vi "Autonomous Independent.vi"   [LabVIEW 2013]
doc: "This VI is called when autonomous begins, and will automatically be terminated when autonomous ends. You can carry out timed or sensor driven robot movement independently without needing to return to the caller."
uses:
  <vilib>/Rock Robotics/WPI/Solenoid/WPI_SolenoidValue.ctl
  Robot Global Data.vi
  <vilib>/Rock Robotics/WPI/Solenoid/Deprecated/WPI_SolenoidGetBool.vi
  <vilib>/Rock Robotics/WPI/Solenoid/WPI_SolenoidSetEnum.vi
  <vilib>/Rock Robotics/WPI/RobotDrive/WPI_RobotDriveGetSetRefNum.vi
  <vilib>/Rock Robotics/WPI/RobotDrive/WPI_RobotDriveArcadeDrive_Standard(NoSaturation).vi
  <vilib>/Rock Robotics/WPI/Joystick/WPI_JoystickGetSetRefNum.vi
panel:
  # "Be sure to right-click and choose Data Operations>>Make Current Value default if you want to save the array values with the VI"
types:
  T1 = typedef "WPI_JoystickDevRef.ctl" = cluster{"Device":T2}
  T2 = typedef "WPI_JoystickDeviceEnum.ctl" = enum16{"USB 1", "USB 2", "USB 3", "USB 4", "Kinect 1", "Kinect 2"}
  T3 = typedef "WPI_SolenoidDevRef.ctl" = cluster{"DevStatus":errorcluster, "Solenoid Module":T4, "Forward Solenoid Channel":T5, "Reverse Solenoid Channel":T5}
  T4 = typedef "FPGA_TypedefSolenoidModule.ctl" = enum16{"Solenoid Module 1", "Solenoid Module 2"}
  T5 = typedef "WPI_SolenoidChannel.ctl" = enum8{"Solenoid 1", "Solenoid 2", "Solenoid 3", "Solenoid 4", "Solenoid 5", "Solenoid 6", "Solenoid 7", "Solenoid 8", "Invalid"}
  T6 = typedef "WPI_SolenoidValue.ctl" = enum16{"Off", "On", "Forward", "Reverse"}
  T7 = typedef "WPI_RobotDriveDevRef.ctl" = cluster{"DevStatus":errorcluster, "Motors[]":T8[], "Square Inputs":bool, "Max Output":dbl, "Isochronous":bool}
  T8 = typedef "WPI_MotorControlDeviceRef.ctl" = cluster{"DeviceStatus":errorcluster, "Type":enum16{"PWM", "CAN"}, "PWM":cluster{"Digital Module":T9, "PWM Channel":T10, "DeadBand":T11}, "CAN":cluster{"Device Number":u8, "Control Mode":T12, "Semaphore":T13, "Max Vout":dbl}, "Invert":bool, "TransformRef":T14, "InvTransformRef":T14}
  T9 = typedef "FPGA_TypedefDigitalModule.ctl" = enum16{"Digital Module 1", "Digital Module 2"}
  T10 = typedef "FPGA_DIOPWMChannel.ctl" = enum8{"PWM 1", "PWM 2", "PWM 3", "PWM 4", "PWM 5", "PWM 6", "PWM 7", "PWM 8", "PWM 9", "PWM 10", "Invalid"}
  T11 = typedef "WPI_PWMDeadband.ctl" = cluster{"Name":string, "maxPositivePwm":i32, "minPositivePwm":i32, "centerPwm":i32, "maxNegativePwm":i32, "minNegativePwm":i32, "angularRange":u16}
  T12 = typedef "WPI_CANJaguar_ControlMode.ctl" = enum8{"Percent VBus", "Current", "Speed", "Position", "Voltage"}
  T13 = typedef "Semaphore RefNum" = refnum<k1>
  T14 = typedef "WPI_PWMTransform_ConPane.ctl" = refnum<vi>
  T15 = cluster{"axis 1 (x)":dbl, "axis 2 (y)":dbl, "axis 3 (throttle)":dbl, "axis 4":dbl, "axis 5":dbl, "axis 6":dbl}
  T16 = typedef "WPI_DigitalInputDevRef.ctl" = cluster{"DevStatus":errorcluster, "DIO Channel":T17, "Digital Module":T9}
  T17 = typedef "FPGA_DIOChannel.ctl" = enum8{"DIO 1", "DIO 2", "DIO 3", "DIO 4", "DIO 5", "DIO 6", "DIO 7", "DIO 8", "DIO 9", "DIO 10", "DIO 11", "DIO 12", "DIO 13", "DIO 14", "Invalid"}
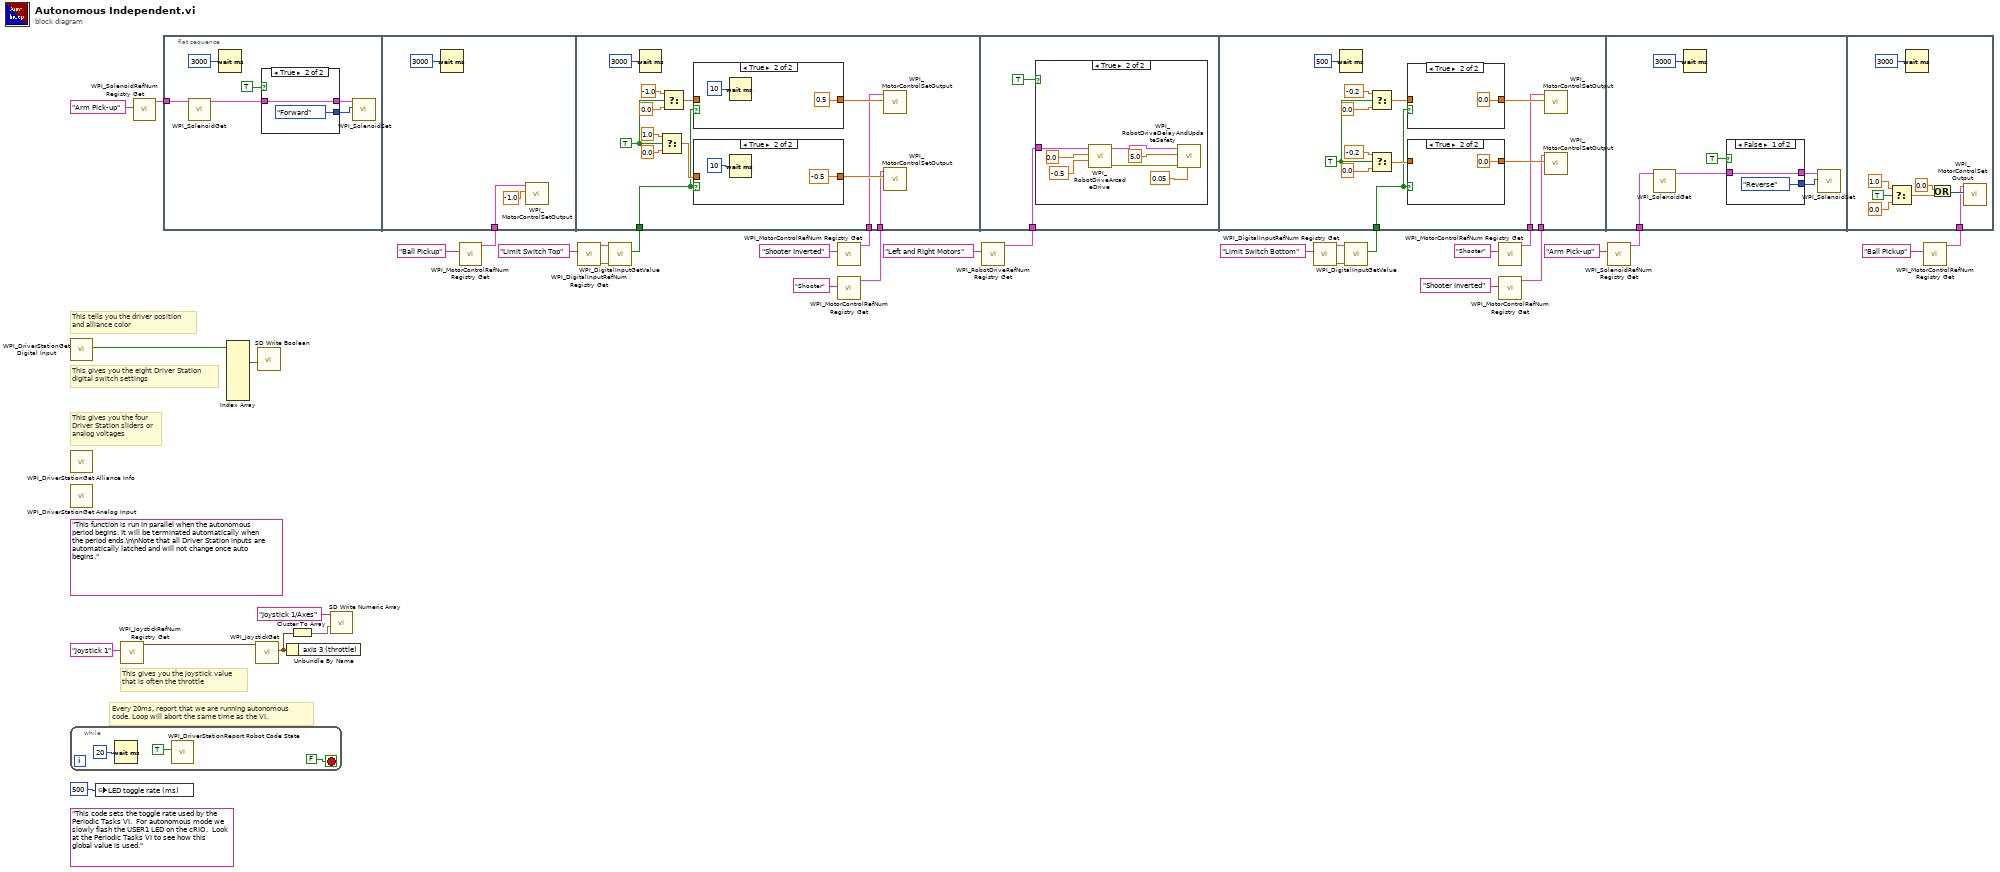
[diagram p0: block diagram]
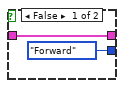
[diagram p2: hidden frame]
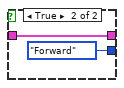
[diagram p8: hidden frame]
diagram:
  (unwired) "This code sets the toggle rate used by the Periodic Tasks VI.  For autonomous mode we slowly flash the USER1 LED on the cRIO.  Look at the Periodic Tasks VI to see how this global value is used."
  (unwired) "This function is run in parallel when the autonomous period begins. It will be terminated automatically when the period ends.\n\nNote that all Driver Station inputs are automatically latched and will not change once auto begins."
  # "Every 20ms, report that we are running autonomous\ncode. Loop will abort the same time as the VI."
  # "This gives you the joystick value\nthat is often the throttle"
  # "This tells you the driver position\nand alliance color"
  # "This gives you the eight Driver Station\ndigital switch settings"
  # "This gives you the four\nDriver Station sliders or\nanalog voltages"
  n1 = call <vilib>:"WPI_DriverStationGet Digital Input.vi"() -> ("Driver Station Digital Input (1-8)"=w34:bool[])  [unwired: 11 out]
  n2 = call <vilib>:"WPI_DriverStationGet Alliance Info.vi"() -> ()  [unwired: 12 out]
  n3 = call <vilib>:"WPI_DriverStationGet Analog Input.vi"() -> ()  [unwired: 12 out]
  n4 = while {
    stop <- FALSE stop-if-true
    n5 = Wait (ms)(milliseconds to wait=u32 20) -> ()  [unwired: 1 out]
    n6 = call <vilib>:"WPI_DriverStationReport Robot Code State.vi"("Autonomous"=TRUE) -> ()  [unwired: 10 in, 1 out]
  }
  n7 = global write "Robot Global Data.vi" "LED toggle rate (ms)"(u32 500 ("LED ms toggle rate")) -> ()
  n8 = call <vilib>:"WPI_JoystickRefNum Registry Get.vi"("refnum name"="Joystick 1") -> ("JoystickDevRef"=w32:T1)  [unwired: 1 in, 9 out]
  n9 = call <vilib>:"WPI_SolenoidRefNum Registry Get.vi"("refnum name"="Arm Pick-up") -> ("SolenoidDevRef"=w9:T3)  [unwired: 9 in, 1 out]
  n10 = flat-sequence {
    tunnel: w9 -> [w38]
    tunnel: w15 -> [w49]
    tunnel: w18 -> [w53]
    tunnel: w13 -> [w52]
    tunnel: w11 -> [w51]
    tunnel: w17 -> [w70]
    tunnel: w22 -> [w81]
    tunnel: w7 -> [w80]
    tunnel: w5 -> [w79]
    tunnel: w3 -> [w96]
    tunnel: w1 -> [w106]
    frame #0 {
      n11 = call-poly <vilib>:"WPI_SolenoidGet.vi"("SolenoidDevRef"=w38) -> ("SolenoidDevRef"=w43:T3)  [unwired: 8 in, 2 out]
      n12 = Wait (ms)(milliseconds to wait=u32 3000) -> ()  [unwired: 1 out]
      n13 = case shown="True" TRUE {
        tunnel: w43 -> [w44 w47]
        tunnel: [w44 w47] -> w42
        tunnel: [WPI_SolenoidValue."Forward" ("Value") WPI_SolenoidValue."Forward" ("Value")] -> w41
        frame False {
        }
        frame True {
        }
      }
      n14 = call-poly <vilib>:"WPI_SolenoidSet.vi"("Value"=w41, "SolenoidDevRef"=w42) -> ()  [unwired: 8 in, 2 out]
    }
    frame #1 {
      n15 = Wait (ms)(milliseconds to wait=u32 3000) -> ()  [unwired: 1 out]
      n16 = call <vilib>:"WPI_MotorControlSetOutput.vi"("Output"=-1.0, "MotorControlDevRef"=w49) -> ()  [unwired: 7 in, 3 out]
    }
    frame #2 {
      w57 = TRUE
      n17 = Wait (ms)(milliseconds to wait=u32 3000) -> ()  [unwired: 1 out]
      n18 = Select(t=1.0, s=w57, f=0.0) -> (s? t:f=w63:dbl)
      n19 = Select(t=-1.0, s=w57, f=0.0) -> (s? t:f=w60:dbl)
      n20 = case shown="True" w53 {
        tunnel: [w64 0.5 ("f")] -> w58
        tunnel: w60 -> [w64 _]
        frame False {
        }
        frame True {
          n21 = Wait (ms)(milliseconds to wait=u32 10) -> ()  [unwired: 1 out]
        }
      }
      n22 = case shown="True" w53 {
        tunnel: [w67 -0.5 ("f")] -> w61
        tunnel: w63 -> [w67 _]
        frame False {
        }
        frame True {
          n23 = Wait (ms)(milliseconds to wait=u32 10) -> ()  [unwired: 1 out]
        }
      }
      n24 = call <vilib>:"WPI_MotorControlSetOutput.vi"("Output"=w58, "MotorControlDevRef"=w52) -> ()  [unwired: 7 in, 3 out]
      n25 = call <vilib>:"WPI_MotorControlSetOutput.vi"("Output"=w61, "MotorControlDevRef"=w51) -> ()  [unwired: 7 in, 3 out]
    }
    frame #3 {
      n26 = case shown="True" TRUE {
        tunnel: w70 -> [_ w78]
        frame False {
        }
        frame True {
          n27 = call-poly <vilib>:"WPI_RobotDriveArcadeDrive.vi"("Y axis value"=-0.5, "X axis value"=0.0, "RobotDriveDevRef"=w78) -> ("error out"=w75:errorcluster, "RobotDriveDevRef"=w74:T7)  [unwired: 6 in, 1 out]
          n28 = call <vilib>:"WPI_RobotDriveDelayAndUpdateSafety.vi"("Feed time (s)"=0.05, "error in (no error)"=w75, "Delay (s)"=5.0, "RobotDriveDevRef"=w74) -> ()  [unwired: 6 in, 2 out]
        }
      }
    }
    frame #4 {
      w82 = TRUE
      n29 = Wait (ms)(milliseconds to wait=u32 500) -> ()  [unwired: 1 out]
      n30 = Select(t=-0.2, s=w82, f=0.0) -> (s? t:f=w84:dbl)
      n31 = Select(t=-0.2, s=w82, f=0.0) -> (s? t:f=w83:dbl)
      n32 = case shown="True" w81 {
        tunnel: [w94 0.0 ("f")] -> w89
        tunnel: w84 -> [w94 _]
        frame False {
        }
        frame True {
        }
      }
      n33 = case shown="True" w81 {
        tunnel: [w92 0.0 ("f")] -> w86
        tunnel: w83 -> [w92 _]
        frame False {
        }
        frame True {
        }
      }
      n34 = call <vilib>:"WPI_MotorControlSetOutput.vi"("Output"=w89, "MotorControlDevRef"=w79) -> ()  [unwired: 7 in, 3 out]
      n35 = call <vilib>:"WPI_MotorControlSetOutput.vi"("Output"=w86, "MotorControlDevRef"=w80) -> ()  [unwired: 7 in, 3 out]
    }
    frame #5 {
      n36 = call-poly <vilib>:"WPI_SolenoidGet.vi"("SolenoidDevRef"=w96) -> ("SolenoidDevRef"=w101:T3)  [unwired: 8 in, 2 out]
      n37 = Wait (ms)(milliseconds to wait=u32 3000) -> ()  [unwired: 1 out]
      n38 = case shown="False" TRUE {
        tunnel: w101 -> [w102 w105]
        tunnel: [w102 w105] -> w100
        tunnel: [WPI_SolenoidValue."Reverse" ("Value") WPI_SolenoidValue."Forward" ("Value")] -> w99
        frame False {
        }
        frame True {
        }
      }
      n39 = call-poly <vilib>:"WPI_SolenoidSet.vi"("Value"=w99, "SolenoidDevRef"=w100) -> ()  [unwired: 8 in, 2 out]
    }
    frame #6 {
      n40 = Select(t=1.0, s=TRUE, f=0.0) -> (s? t:f=w110:dbl)
      n41 = Wait (ms)(milliseconds to wait=u32 3000) -> ()  [unwired: 1 out]
      n42 = Or(x=0.0, y=w110) -> (x .or. y?=w109:i32)
      n43 = call <vilib>:"WPI_MotorControlSetOutput.vi"("Output"=w109, "MotorControlDevRef"=w106) -> ()  [unwired: 7 in, 3 out]
    }
  }
  n44 = Index Array(array=w34) -> (element #2=w27:bool)  [unwired: 8 in, 7 out]
  n45 = call <vilib>:"WPI_JoystickGet.vi"("JoystickDevRef"=w32) -> ("Axes"=w29:T15)  [unwired: 1 in, 5 out]
  n46 = call <vilib>:"SD Write Boolean.vi"("Boolean"=w27) -> ()  [unwired: 9 in, 2 out]
  n47 = Unbundle By Name(w29) -> ()  [unwired: 1 out]
  n48 = Cluster To Array(cluster=w29) -> (array=w30:dbl[])
  n49 = call <vilib>:"SD Write Numeric Array.vi"("Numeric Array"=w30, "Name"="Joystick 1/Axes") -> ()  [unwired: 8 in, 2 out]
  n50 = call <vilib>:"WPI_MotorControlRefNum Registry Get.vi"("refnum name"="Ball Pickup") -> ("MotorControlDevRef"=w15:T8)  [unwired: 9 in, 1 out]
  n51 = call <vilib>:"WPI_DigitalInputRefNum Registry Get.vi"("refnum name"="Limit Switch Top") -> ("error out"=w20:errorcluster, "DigitalInputDevRef"=w21:T16)  [unwired: 9 in]
  n52 = call <vilib>:"WPI_DigitalInputGetValue.vi"("error in (no error)"=w20, "DigitalInputDevRef"=w21) -> ("Value"=w18:bool)  [unwired: 7 in, 2 out]
  n53 = call <vilib>:"WPI_MotorControlRefNum Registry Get.vi"("refnum name"="Shooter Inverted") -> ("MotorControlDevRef"=w13:T8)  [unwired: 9 in, 1 out]
  n54 = call <vilib>:"WPI_MotorControlRefNum Registry Get.vi"("refnum name"="Shooter") -> ("MotorControlDevRef"=w11:T8)  [unwired: 9 in, 1 out]
  n55 = call <vilib>:"WPI_RobotDriveRefNum Registry Get.vi"("refnum name"="Left and Right Motors") -> ("RobotDriveDevRef"=w17:T7)  [unwired: 9 in, 1 out]
  n56 = call <vilib>:"WPI_DigitalInputRefNum Registry Get.vi"("refnum name"="Limit Switch Bottom") -> ("error out"=w24:errorcluster, "DigitalInputDevRef"=w25:T16)  [unwired: 9 in]
  n57 = call <vilib>:"WPI_DigitalInputGetValue.vi"("error in (no error)"=w24, "DigitalInputDevRef"=w25) -> ("Value"=w22:bool)  [unwired: 7 in, 2 out]
  n58 = call <vilib>:"WPI_MotorControlRefNum Registry Get.vi"("refnum name"="Shooter") -> ("MotorControlDevRef"=w5:T8)  [unwired: 9 in, 1 out]
  n59 = call <vilib>:"WPI_MotorControlRefNum Registry Get.vi"("refnum name"="Shooter Inverted") -> ("MotorControlDevRef"=w7:T8)  [unwired: 9 in, 1 out]
  n60 = call <vilib>:"WPI_SolenoidRefNum Registry Get.vi"("refnum name"="Arm Pick-up") -> ("SolenoidDevRef"=w3:T3)  [unwired: 9 in, 1 out]
  n61 = call <vilib>:"WPI_MotorControlRefNum Registry Get.vi"("refnum name"="Ball Pickup") -> ("MotorControlDevRef"=w1:T8)  [unwired: 9 in, 1 out]
